vi "Get Short Name.vi"(8 "error in (no error)":errorcluster, 11 "Analyze Results Base in":refnum<class "Analyze Results Base.lvclass">) -> (0 "error out":errorcluster, 2 "Short Name":string, 3 "Analyze Results Base out":refnum<class "Analyze Results Base.lvclass">)   [LabVIEW 2020, in "Analyze Results Base.lvclass"]
uses:
  Analyze Results Base.lvclass
  Analyze Results Base.lvclass/Analyze Results Base.ctl
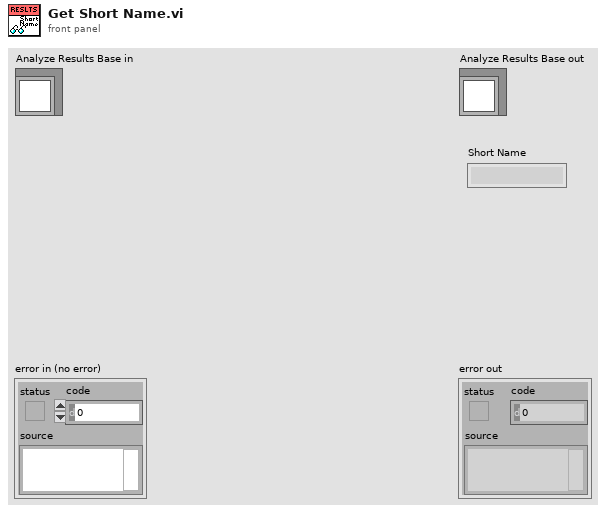
[diagram p1: front panel]
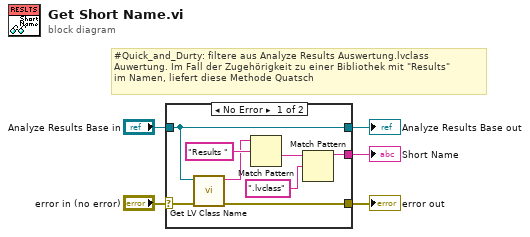
[diagram p0: block diagram]
diagram:
  # "#Quick_and_Durty: filtere aus Analyze Results Auswertung.lvclass\nAuwertung. Im Fall der Zugehörigkeit zu einer Bibliothek mit \"Results\" \nim Namen, liefert diese Methode Quatsch"
  n1 = case shown="No Error" "error in (no error)" {
    selector: "error in (no error)" -> [w7 w15]
    tunnel: [w6 w15] -> w4
    tunnel: [w10 w14] -> w2
    tunnel: "Analyze Results Base in" -> [w10 w14]
    tunnel: [w8 _] -> w1
    frame No Error {
      n2 = call <vilib>:"Get LV Class Name.vi"("error in (no error)"=w7, "object"=w10) -> ("error out"=w6:errorcluster, "class name"=w9:string)  [unwired: 8 in]
      n3 = Match Pattern(string=w9, regular expression="Results ") -> (after substring=w11:string)  [unwired: 1 in, 3 out]
      n4 = Match Pattern(string=w11, regular expression=".lvclass") -> (before substring=w8:string)  [unwired: 1 in, 3 out]
    }
    frame Error {
    }
  }
  "error out" <- w4
  "Analyze Results Base out" <- w2
  "Short Name" <- w1
